vi "psition_winkel_zu_text.vi"(9 "X":dbl, 10 "Y":dbl, 11 "Angle":sgl) -> (3 "String":string)   [LabVIEW 2014]
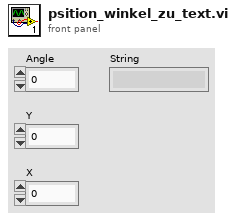
[diagram p1: front panel]
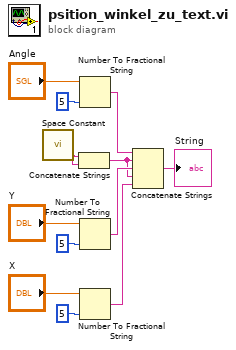
[diagram p0: block diagram]
diagram:
  n1 = call <vilib>:"Space Constant.vi"() -> ("String"=w7:string)
  n2 = Concatenate Strings(w7, w7) -> (w8:string)
  n3 = Number To Fractional String(number="Angle", precision (6)=i16 5) -> (F-format string=w9:string)  [unwired: 2 in]
  n4 = Number To Fractional String(number="Y", precision (6)=i16 5) -> (F-format string=w10:string)  [unwired: 2 in]
  n5 = Number To Fractional String(number="X", precision (6)=i16 5) -> (F-format string=w11:string)  [unwired: 2 in]
  n6 = Concatenate Strings(w9, w8, w10, w8, w11) -> (→"String":string)
